vi "ESP Simple Front Panel for RS232.vi"() -> ()   [LabVIEW 2017]
panel:
  in  "Exit":bool
  in  "COM Port":T1(ring)
  in  "Relative Move":dbl format="%.3f"
  in  "Move Rel.":bool
  in  "Velocity (mm/s)":dbl=1.0 format="%.3f"
  in  "Set":bool
  in  "Motor OFF":bool
  in  "Axis":i32=1 min=1 max=6
  in  "Target position":dbl format="%.3f"
  in  "Move":bool
  in  "Get position":bool
  in  "Motor ON":bool
  out "Position status":dbl format="%.3f"
  # "Set COM port before starting vi"
  # "Communication is set for Com1 and default ESP controller settings.\nTo make changes, modify the appropriate parameters on the wiring diagram."
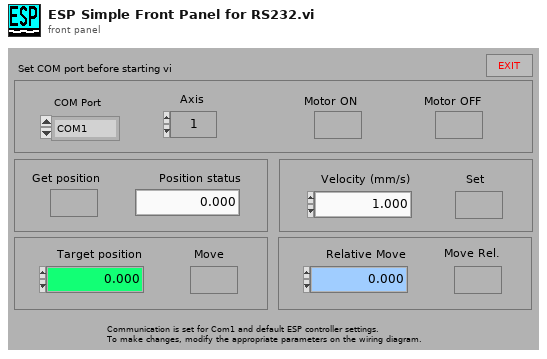
[diagram p1: front panel]
types:
  T1 = enum16{"COM1", "COM2", "COM3", "COM4", "COM5", "COM6", "COM7", "COM8", "COM9"}
  T2 = cluster{"input XON/XOFF":bool, "input HW Handshake":bool, "input alt HW HShk":bool, "output XON/XOFF":bool, "output HW Handshake":bool, "output alt HW HShk":bool, "XOFF byte":u8, "XON byte":u8, "parity error byte":u16}
  T3 = enum16{"no parity", "odd parity", "even parity", "mark parity", "space parity"}
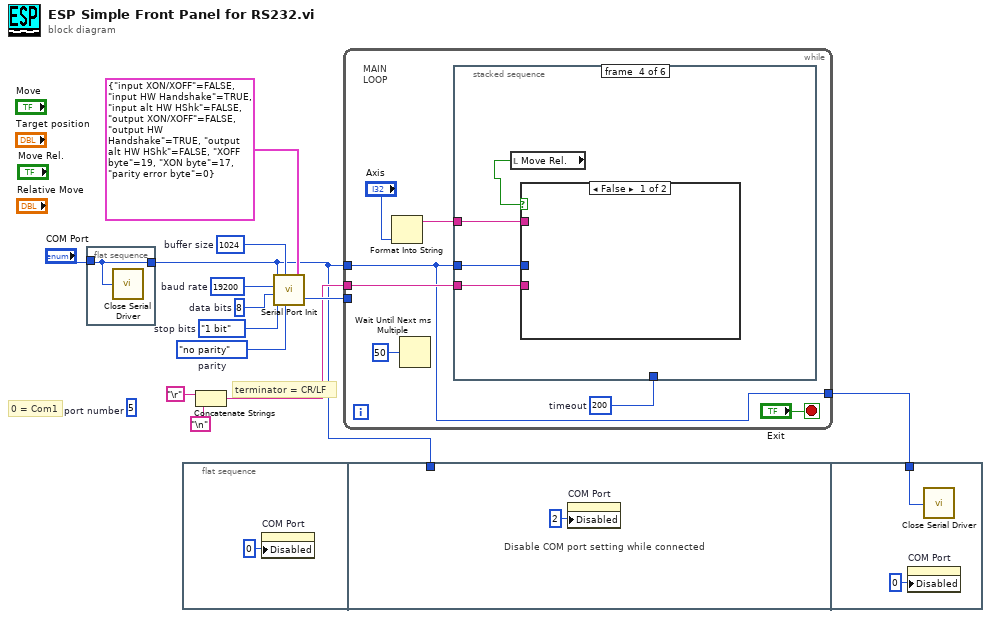
[diagram p0: block diagram]
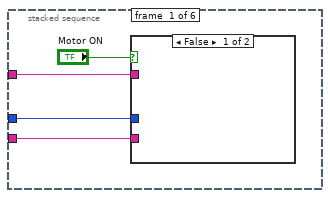
[diagram p2: hidden frame]
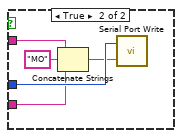
[diagram p3: hidden frame]
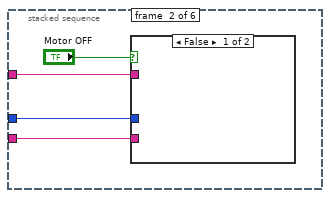
[diagram p4: hidden frame]
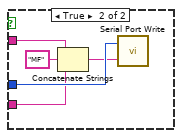
[diagram p5: hidden frame]
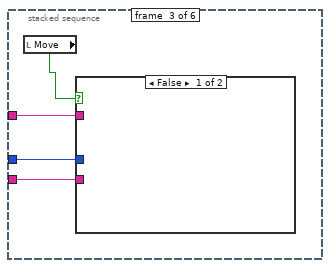
[diagram p6: hidden frame]
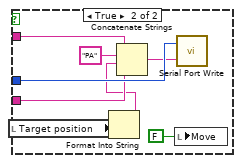
[diagram p7: hidden frame]
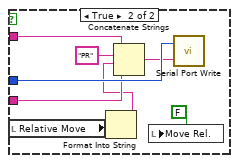
[diagram p8: hidden frame]
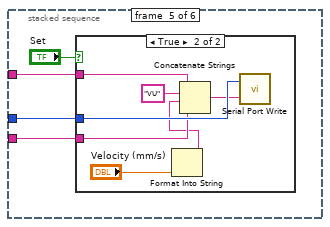
[diagram p9: hidden frame]
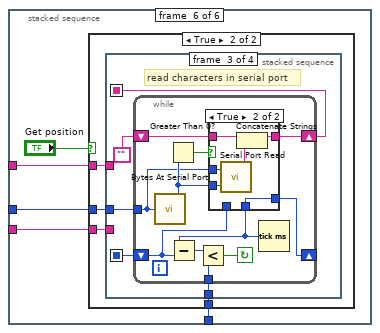
[diagram p11: hidden frame]
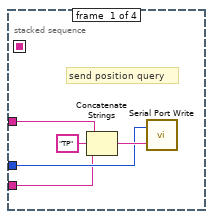
[diagram p13: hidden frame]
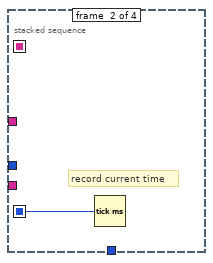
[diagram p14: hidden frame]
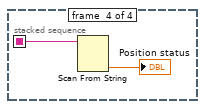
[diagram p16: hidden frame]
diagram:
  w9 = u32 19200  # baud rate
  w10 = u16 8  # data bits
  w11 = enum16{"1 bit", "1.5 bits", "2 bits"}."1 bit"  # stop bits
  w12 = T3."no parity"  # parity
  (unwired) 5  # port number
  w13 = u16 1024  # buffer size
  # "terminator = CR/LF"
  # "0 = Com1"
  n1 = flat-sequence {
    tunnel: "COM Port" -> [w14]
    tunnel: [w14] -> w1
    frame #0 {
      n2 = call <vilib>:"Close Serial Driver.vi"("port number"=w14) -> ()  [unwired: 1 out]
    }
  }
  n3 = flat-sequence {
    tunnel: w1 -> [_]
    tunnel: w3 -> [w17]
    frame #0 {
      n4 = property on="COM Port" class="Enum (strict)"("Disabled"=u8 0) -> ()  [unwired: 2 in, 2 out]
    }
    frame #1 {
      # "Disable COM port setting while connected"
      n5 = property on="COM Port" class="Enum (strict)"("Disabled"=u8 2) -> ()  [unwired: 2 in, 2 out]
    }
    frame #2 {
      n6 = property on="COM Port" class="Enum (strict)"("Disabled"=u8 0) -> ()  [unwired: 2 in, 2 out]
      n7 = call <vilib>:"Close Serial Driver.vi"("port number"=w17) -> ()  [unwired: 1 out]
    }
  }
  n8 = Concatenate Strings("\r", "\n") -> (w4:string)
  n9 = call <vilib>:"Serial Port Init.vi"("flow control etc."=T2 {"input XON/XOFF"=FALSE, "input HW Handshake"=TRUE, "input alt HW HShk"=FALSE, "output XON/XOFF"=FALSE, "output HW Handshake"=TRUE, "output alt HW HShk"=FALSE, "XOFF byte"=19, "XON byte"=17, "parity error byte"=0}, "parity"=w12, "buffer size"=w13, "stop bits"=w11, "data bits"=w10, "baud rate"=w9, "port number"=w1) -> ("error code"=w7:i32)
  n10 = while {
    tunnel: w1 -> [w20]
    tunnel: w4 -> [w22]
    tunnel: w7 -> [_]
    tunnel: [w20] -> w3
    stop <- "Exit" stop-if-true
    w21 = u32 200  # timeout
    # "MAIN\nLOOP"
    n11 = Format Into String("Axis") -> (resulting string=w23:string)  [unwired: 3 in, 1 out]
    n12 = Wait Until Next ms Multiple(millisecond multiple=u32 50) -> ()  [unwired: 1 out]
    n13 = stacked-sequence {
      tunnel: w23 -> [w27 w37 w46 w58 w70 w82]
      tunnel: w22 -> [w26 w36 w45 w57 w69 w79]
      tunnel: w20 -> [w28 w38 w47 w59 w71 w81]
      tunnel: w21 -> [_ _ _ _ _ w80]
      frame #0 {
        n14 = case shown="False" "Motor ON" {
          tunnel: w28 -> [_ w34]
          tunnel: w27 -> [_ w31]
          tunnel: w26 -> [_ w30]
          frame False {
          }
          frame True {
            n15 = Concatenate Strings(w31, "MO" ("Substring"), w30) -> (w32:string)
            n16 = call <vilib>:"Serial Port Write.vi"("string to write"=w32, "port number"=w34) -> ()  [unwired: 1 out]
          }
        }
      }
      frame #1 {
        n17 = case shown="False" "Motor OFF" {
          tunnel: w38 -> [_ w43]
          tunnel: w37 -> [_ w40]
          tunnel: w36 -> [_ w39]
          frame False {
          }
          frame True {
            n18 = Concatenate Strings(w40, "MF" ("Substring"), w39) -> (w41:string)
            n19 = call <vilib>:"Serial Port Write.vi"("string to write"=w41, "port number"=w43) -> ()  [unwired: 1 out]
          }
        }
      }
      frame #2 {
        n20 = local read "Move"() -> (w44:bool)
        n21 = case shown="False" w44 {
          tunnel: w47 -> [_ w55]
          tunnel: w46 -> [_ w52]
          tunnel: w45 -> [_ w51]
          frame False {
          }
          frame True {
            n22 = local read "Target position"() -> (w49:dbl)
            n23 = Format Into String(w49) -> (resulting string=w50:string)  [unwired: 3 in, 1 out]
            n24 = Concatenate Strings(w52, "PA" ("Substring"), w50, w51) -> (w53:string)
            n25 = local write "Move"(FALSE ("Move")) -> ()
            n26 = call <vilib>:"Serial Port Write.vi"("string to write"=w53, "port number"=w55) -> ()  [unwired: 1 out]
          }
        }
      }
      frame #3 {
        n27 = local read "Move Rel."() -> (w56:bool)
        n28 = case shown="False" w56 {
          tunnel: w59 -> [_ w67]
          tunnel: w58 -> [_ w64]
          tunnel: w57 -> [_ w63]
          frame False {
          }
          frame True {
            n29 = local read "Relative Move"() -> (w61:dbl)
            n30 = Format Into String(w61) -> (resulting string=w62:string)  [unwired: 3 in, 1 out]
            n31 = Concatenate Strings(w64, "PR" ("Substring"), w62, w63) -> (w65:string)
            n32 = local write "Move Rel."(FALSE ("Move Rel.")) -> ()
            n33 = call <vilib>:"Serial Port Write.vi"("string to write"=w65, "port number"=w67) -> ()  [unwired: 1 out]
          }
        }
      }
      frame #4 {
        n34 = case shown="True" "Set" {
          tunnel: w71 -> [_ w78]
          tunnel: w70 -> [_ w75]
          tunnel: w69 -> [_ w74]
          frame False {
          }
          frame True {
            n35 = Format Into String("Velocity (mm/s)") -> (resulting string=w72:string)  [unwired: 3 in, 1 out]
            n36 = Concatenate Strings(w75, "VU" ("Substring"), w72, w74) -> (w76:string)
            n37 = call <vilib>:"Serial Port Write.vi"("string to write"=w76, "port number"=w78) -> ()  [unwired: 1 out]
          }
        }
      }
      frame #5 {
        n38 = case shown="True" "Get position" {
          tunnel: w82 -> [_ w87]
          tunnel: w81 -> [_ w86]
          tunnel: w80 -> [_ w85]
          tunnel: w79 -> [_ w84]
          frame False {
          }
          frame True {
            n39 = stacked-sequence {
              seq-local: [_ w93 _ _] -> [_ _ w95 _]
              seq-local: [_ _ w94 _] -> [_ _ _ w119]
              tunnel: w87 -> [w90 _ _ _]
              tunnel: w86 -> [w89 _ w98 _]
              tunnel: w85 -> [_ _ w96 _]
              tunnel: w84 -> [w88 _ _ _]
              frame #0 {
                # "send position query"
                n40 = Concatenate Strings(w90, "TP" ("Substring"), w88) -> (w91:string)
                n41 = call <vilib>:"Serial Port Write.vi"("string to write"=w91, "port number"=w89) -> ()  [unwired: 1 out]
              }
              frame #1 {
                # "record current time"
                n42 = Tick Count (ms)() -> (millisecond timer value=w93:u32)
              }
              frame #2 {
                # "read characters in serial port"
                n43 = while {
                  shift-left: w95 -> [w99]
                  shift-right: [w100] -> _
                  tunnel: w96 -> [w103]
                  shift-left: "" -> [w106]
                  shift-right: [w105] -> w94
                  tunnel: w98 -> [w107]
                  stop <- w102 continue-if-true
                  n44 = call <vilib>:"Bytes At Serial Port.vi"("port number"=w107) -> ("byte count"=w108:u32)  [unwired: 1 out]
                  n45 = Greater Than 0?(x=w108) -> (x > 0?=w109:bool)
                  n46 = Tick Count (ms)() -> (millisecond timer value=w101:u32)
                  n47 = Subtract(x=w101, y=w99) -> (x-y=w104:u32)
                  n48 = Less?(x=w104, y=w103) -> (x < y?=w102:bool)
                  n49 = case shown="True" w109 {
                    tunnel: w108 -> [_ w117]
                    tunnel: w107 -> [_ w116]
                    tunnel: w106 -> [w111 w114]
                    tunnel: [w111 w113] -> w105
                    tunnel: [w110 w112] -> w100
                    tunnel: w101 -> [_ w112]
                    tunnel: w99 -> [w110 _]
                    frame False {
                    }
                    frame True {
                      n50 = call <vilib>:"Serial Port Read.vi"("requested byte count"=w117, "port number"=w116) -> ("string read"=w115:string)  [unwired: 1 out]
                      n51 = Concatenate Strings(w114, w115) -> (w113:string)
                    }
                  }
                }
              }
              frame #3 {
                n52 = Scan From String(input string=w119) -> (output 1=→"Position status":dbl)  [unwired: 4 in, 3 out]
              }
            }
          }
        }
      }
    }
  }
